vi "search2DArray.vi"(8 "error in (no error)":errorcluster, 9 "1DArrayToBeSearched":dbl[](array[numeric]), 10 "2DArray":dbl[][](array[numeric]), 11 "Utilities in":refnum<class "Utilities.lvclass">) -> (0 "error out":errorcluster, 1 "firstIndexOfSearched1DArray":i32, 2 "found?":bool, 3 "Utilities out":refnum<class "Utilities.lvclass">)   [LabVIEW 2021, in "Utilities.lvclass"]
uses:
  Utilities.lvclass
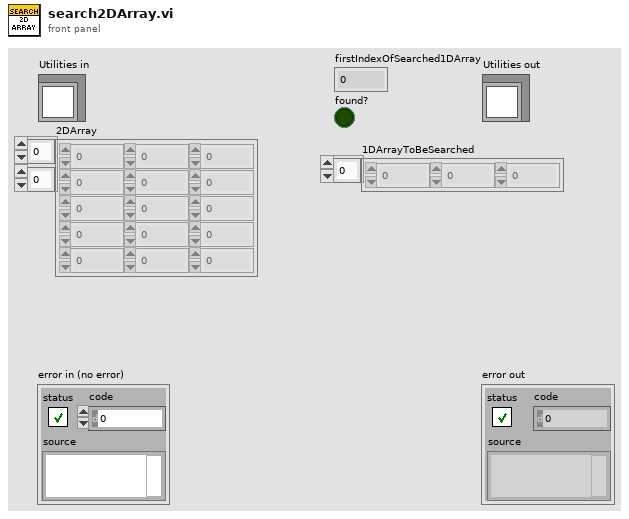
[diagram p1: front panel]
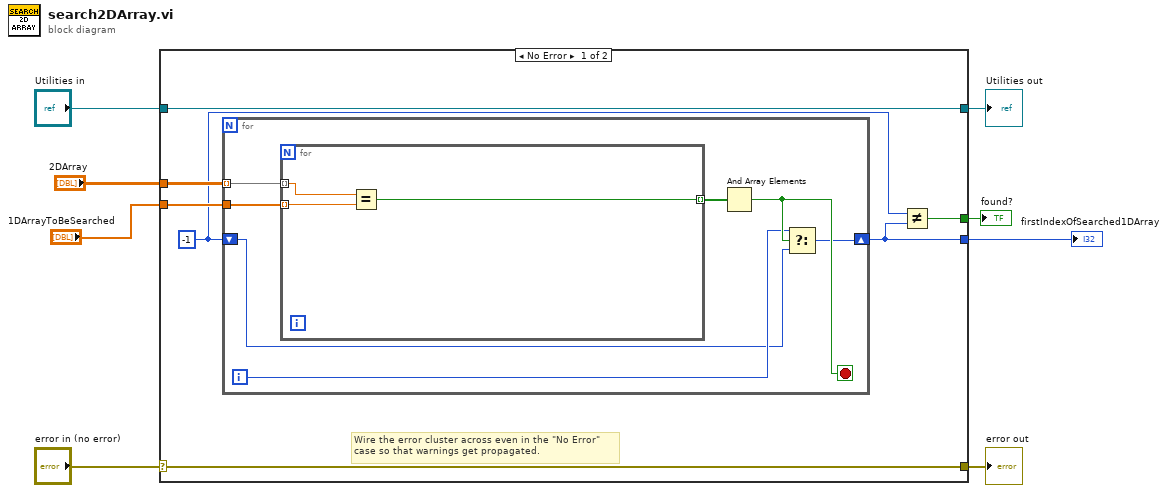
[diagram p0: block diagram]
diagram:
  n1 = case shown="No Error" "error in (no error)" {
    selector: "error in (no error)" -> [w14 w27]
    tunnel: [w14 w27] -> w7
    tunnel: [w15 w26] -> w5
    tunnel: "Utilities in" -> [w15 w26]
    tunnel: "2DArray" -> [w13 _]
    tunnel: "1DArrayToBeSearched" -> [w12 _]
    tunnel: [w11 _] -> w2
    tunnel: [w9 _] -> w1
    frame No Error {
      w10 = -1
      # "Wire the error cluster across even in the \"No Error\"\ncase so that warnings get propagated."
      n2 = for {
        tunnel: w13 -> [w21] mode=indexing
        tunnel: w12 -> [w22]
        shift-right: [w16] -> w11
        shift-left: w10 -> [w17]
        i -> [w18]
        stop <- w19 stop-if-true
        n3 = for {
          tunnel: w22 -> [w25] mode=indexing
          tunnel: w21 -> [w24] mode=indexing
          tunnel: [w23] -> w20 mode=indexing
          n4 = Equal?(x=w24, y=w25) -> (x = y?=w23:bool)
        }
        n5 = And Array Elements(Boolean array=w20) -> (logical AND=w19:bool)
        n6 = Select(t=w18, s=w19, f=w17) -> (s? t:f=w16:i32)
      }
      n7 = Not Equal?(x=w10, y=w11) -> (x != y?=w9:bool)
    }
    frame Error {
    }
  }
  "error out" <- w7
  "Utilities out" <- w5
  "firstIndexOfSearched1DArray" <- w2
  "found?" <- w1
